vi "Get_Angles.vi"(8 "error in (no error)":errorcluster, 10 "Deg?":bool, 11 "reference in":refnum<class "Manipulator.lvclass">) -> (0 "error out":errorcluster, 2 "Angles":T1, 3 "reference out":refnum<class "Manipulator.lvclass">)   [LabVIEW 2014, in "Manipulator.lvclass"]
uses:
  Manipulator.lvclass
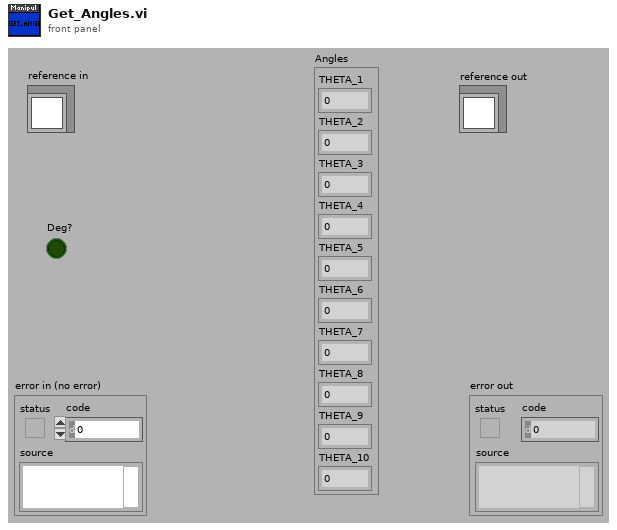
[diagram p1: front panel]
types:
  T1 = cluster{"THETA_1":dbl, "THETA_2":dbl, "THETA_3":dbl, "THETA_4":dbl, "THETA_5":dbl, "THETA_6":dbl, "THETA_7":dbl, "THETA_8":dbl, "THETA_9":dbl, "THETA_10":dbl}
  T2 = typedef "Manipulator.lvclass/ObjectAttributes.ctl" = cluster{"Coordinates":cluster{"X":dbl, "Y":dbl, "Z":dbl}, "Angles":cluster{"THETA_1":dbl, "THETA_2":dbl, "THETA_3":dbl, "THETA_4":dbl, "THETA_5":dbl, "THETA_6":dbl, "THETA_7":dbl, "THETA_8":dbl, "THETA_9":dbl, "THETA_10":dbl}, "Lengths":cluster{"a":dbl, "b":dbl, "c":dbl, "d":dbl, "e":dbl}, "Coordinates of joints":cluster{"A":cluster{"X":dbl, "Y":dbl, "Z":dbl}, "B":cluster{"X":dbl, "Y":dbl, "Z":dbl}, "C":cluster{"X":dbl, "Y":dbl, "Z":dbl}, "D":cluster{"X":dbl, "Y":dbl, "Z":dbl}}}
  T3 = cluster{"[0]":dbl, "[1]":dbl, "[2]":dbl, "[3]":dbl, "[4]":dbl, "[5]":dbl, "[6]":dbl, "[7]":dbl, "[8]":dbl}
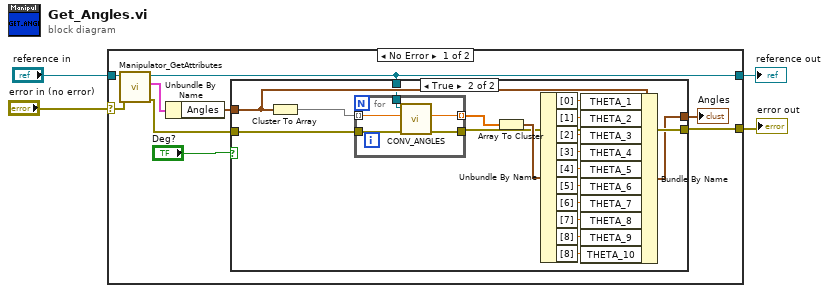
[diagram p0: block diagram]
diagram:
  n1 = case shown="No Error" "error in (no error)" {
    selector: "error in (no error)" -> [w13 w40]
    tunnel: [w8 w40] -> w3
    tunnel: [w6 w39] -> w1
    tunnel: "reference in" -> [w12 w39]
    frame No Error {
      n2 = call "Manipulator_GetAttributes.vi"("error in (no error)"=w13, "reference in"=w12) -> ("error out"=w9:errorcluster, "Data"=w11:T2, "reference out"=w6:refnum<class "Manipulator.lvclass">)  [unwired: 6 in, 1 out]
      n3 = Unbundle By Name(w11) -> ("Angles"=w7:T1)
      n4 = case shown="True" "Deg?" {
        tunnel: w9 -> [w15 w32]
        tunnel: [w14 w17] -> w5
        tunnel: [w15 w28] -> w8
        tunnel: w7 -> [w14 w27]
        tunnel: w6 -> [_ w16]
        frame False {
        }
        frame True {
          n5 = Cluster To Array(cluster=w27) -> (array=w33:dbl[])
          n6 = for {
            tunnel: w33 -> [w36] mode=indexing
            tunnel: w32 -> [w38]
            tunnel: [w37] -> w28
            tunnel: [w35] -> w31 mode=indexing
            tunnel: w16 -> [w34]
            n7 = call "CONV_ANGLES.vi"("error in (no error)"=w38, "IN (RAD)"=w36, "reference in"=w34) -> ("error out"=w37:errorcluster, "OUT (DEG)"=w35:dbl)  [unwired: 5 in, 2 out]
          }
          n8 = Array To Cluster(array=w31) -> (cluster=w30:T3)
          n9 = Unbundle By Name(w30) -> ("[0]"=w29:dbl, "[1]"=w26:dbl, "[2]"=w25:dbl, "[3]"=w24:dbl, "[4]"=w23:dbl, "[5]"=w22:dbl, "[6]"=w21:dbl, "[7]"=w20:dbl, "[8]"=w19:dbl, "[8]"=w18:dbl)
          n10 = Bundle By Name(cluster=w27, "THETA_1"=w29, "THETA_2"=w26, "THETA_3"=w25, "THETA_4"=w24, "THETA_5"=w23, "THETA_6"=w22, "THETA_7"=w21, "THETA_8"=w20, "THETA_9"=w19, "THETA_10"=w18) -> (w17:T1)
        }
      }
      "Angles" <- w5
    }
    frame Error {
    }
  }
  "error out" <- w3
  "reference out" <- w1
